vi "Read Channel Mapping.vi"(8 "error in (no error)":errorcluster) -> ()   [LabVIEW 2017]
uses:
  <vilib>/Utility/file.llb/Read Delimited Spreadsheet (string).vi
  SubVI - Global.vi
panel:
  out "Array":bool[](array[boolean])
  out "all rows":string[][](array[string])
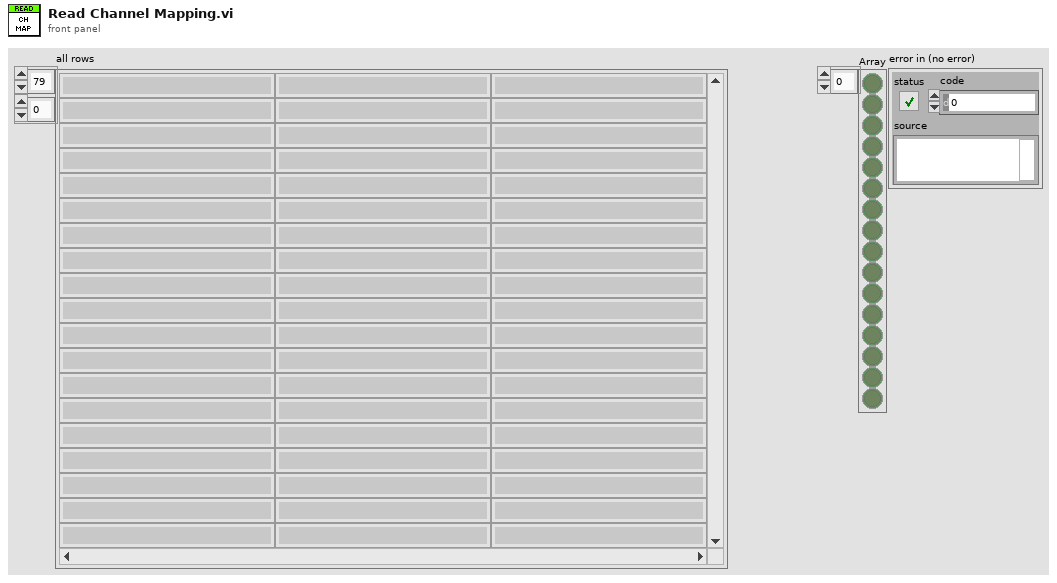
[diagram p1: front panel]
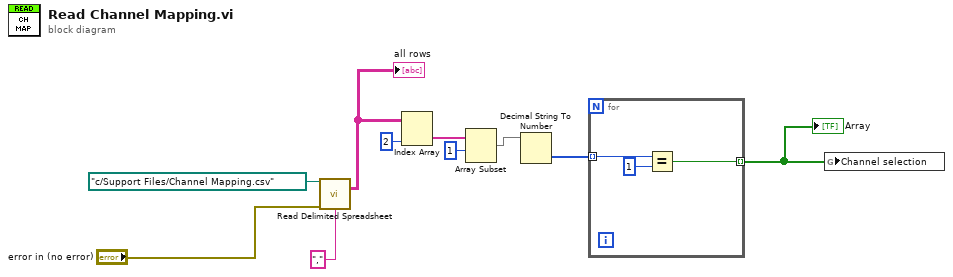
[diagram p0: block diagram]
diagram:
  n1 = call-poly <vilib>:"Read Delimited Spreadsheet.vi"("file path (dialog if empty)"=path "c:/Support Files/Channel Mapping.csv", "error in (no error)"="error in (no error)", "delimiter (\\t)"="," ("delimiter (\\t)")) -> ("all rows"=w9:string[][])  [unwired: 7 in, 5 out]
  "all rows" <- w9
  n2 = Index Array(array=w9, index (col)=2 ("disabled index (col)")) -> (element=w3:string[])  [unwired: 1 in]
  n3 = Array Subset(array=w3, index=1) -> (w2:string[])  [unwired: 1 in]
  n4 = Decimal String To Number(string=w2) -> (number=w7:i32[])  [unwired: 2 in, 1 out]
  n5 = for {
    tunnel: w7 -> [w13] mode=indexing
    tunnel: [w11] -> w6 mode=indexing
    n6 = Equal?(x=w13, y=1) -> (x = y?=w11:bool)
  }
  "Array" <- w6
  n7 = global write "SubVI - Global.vi" "Channel selection"(w6) -> ()
